vi "OCR_FOV.vi"(3 "error in":errorcluster, 4 "Size factor":dbl, 5 "Image in":T1) -> (0 "error out":errorcluster, 1 "FOV":dbl, 2 "Image out":T1(plugin-control))   [LabVIEW 2014]
uses:
  <vilib>/vision/NI_Vision_Development_Module.lvlib
  <vilib>/vision/Image Controls.llb/IMAQ Image.ctl
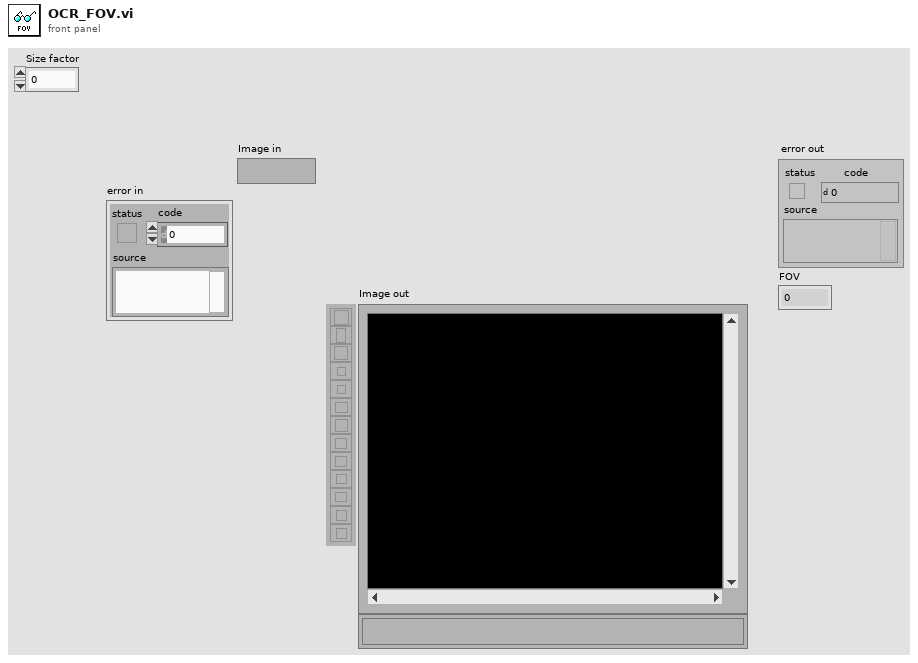
[diagram p1: front panel]
types:
  T1 = typedef "IMAQ Image.ctl" = refnum<image>
  T2 = cluster{"Dark Characters":bool, "Number of Blocks":i32, "Threshold Limits":cluster{"Lower Value":i32, "Upper Value":i32}, "Optimize For Speed":bool, "Perform Bi-modal Calculation":bool}
  T3 = typedef "IMAQ Rectangle" = cluster{"Left":i32, "Top":i32, "Right":i32, "Bottom":i32, "Rotation":dbl}
  T4 = typedef "IMAQ OCR Session.ctl" = refnum<k1>
  T5 = typedef "ROI Descriptor" = cluster{"Global Rectangle":i32[], "Contours":cluster{"ID":enum32{"External", "Internal"}, "Type":u32, "Coordinates":i32[]}[]}
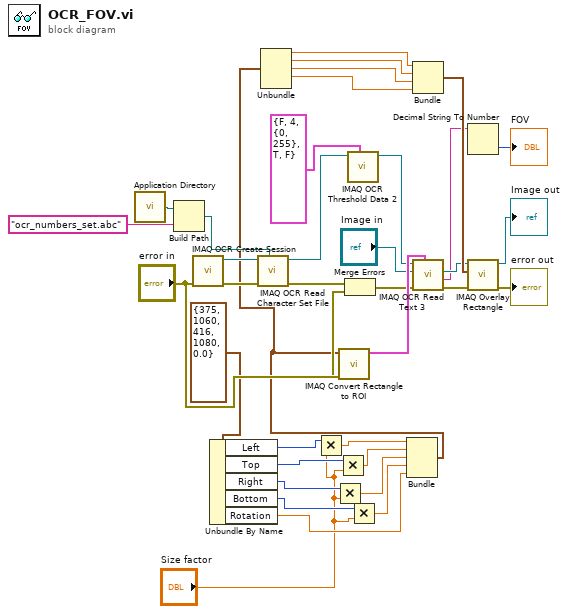
[diagram p0: block diagram]
diagram:
  n1 = call <vilib>:"Application Directory.vi"() -> ("Application Directory"=w25:path)
  n2 = Build Path(base path=w25, name or relative path="ocr_numbers_set.abc") -> (appended path=w23:path)
  n3 = call "IMAQ OCR Create Session"("error in (no error)"="error in") -> ("error out"=w21:errorcluster, "IMAQ OCR Session"=w36:T4)  [unwired: 9 out]
  n4 = Unbundle By Name(T3 {"Left"=375, "Top"=1060, "Right"=416, "Bottom"=1080, "Rotation"=0.0} ("Rectangle")) -> ("Left"=w1:i32, "Top"=w7:i32, "Right"=w12:i32, "Bottom"=w6:i32, "Rotation"=w11:dbl)
  n5 = call "IMAQ OCR Read Character Set File"("File Path"=w23, "error in (no error)"=w21, "IMAQ OCR Session"=w36) -> ("error out"=w20:errorcluster, "IMAQ OCR Session (dup)"=w29:T4)  [unwired: 2 in, 5 out]
  n6 = Multiply(x=w1, y="Size factor") -> (x*y=w2:dbl)
  n7 = Multiply(x=w12, y="Size factor") -> (x*y=w8:dbl)
  n8 = Multiply(x=w7, y="Size factor") -> (x*y=w5:dbl)
  n9 = call-poly "IMAQ OCR Threshold Data 2"("Threshold Data"=T2 {"Dark Characters"=FALSE, "Number of Blocks"=4, "Threshold Limits"={"Lower Value"=0, "Upper Value"=255}, "Optimize For Speed"=TRUE, "Perform Bi-modal Calculation"=FALSE}, "IMAQ OCR Session"=w29) -> ("IMAQ OCR Session (dup)"=w28:T4)  [unwired: 5 in, 4 out]
  n10 = Multiply(x=w6, y="Size factor") -> (x*y=w4:dbl)
  n11 = Bundle(w2, w5, w8, w4, "Rotation"=w11) -> (w9:cluster{dbl, dbl, dbl, dbl, "Rotation":dbl})  [unwired: 1 in]
  n12 = Unbundle(w9) -> (w35:dbl, w34:dbl, w33:dbl, w32:dbl)  [unwired: 1 out]
  n13 = call "IMAQ Convert Rectangle to ROI"("error in (no error)"="error in", "Rectangle"=w9) -> ("error out"=w13:errorcluster, "ROI Descriptor"=w37:T5)  [unwired: 7 in]
  n14 = Merge Errors(w20, w13) -> (w19:errorcluster)
  n15 = Bundle(w35, w34, w33, w32) -> (w31:cluster{dbl, dbl, dbl, dbl})  [unwired: 1 in]
  n16 = call "IMAQ OCR Read Text 3"("ROI Descriptor"=w37, "error in (no error)"=w19, "Image"="Image in", "IMAQ OCR Session"=w28) -> ("error out"=w18:errorcluster, "Read String"=w16:string, "Image (dup)"=w26:T1)  [unwired: 1 in, 4 out]
  n17 = Decimal String To Number(string=w16) -> (number=→"FOV":i32)  [unwired: 2 in, 1 out]
  n18 = call "IMAQ Overlay Rectangle"("error in (no error)"=w18, "Rectangle"=w31, "Image"=w26) -> ("error out"=→"error out":errorcluster, "Image Out"=→"Image out":T1)  [unwired: 7 in]
